vi "variableNames.vi"(11 "pathString":path) -> (2 "spreadsheet string":string, 3 "all rows":string[](array[string]))   [LabVIEW 2017]
uses:
  <userlib>/My Palettes.lib/Files & paths/Spreadsheet/Read From Spreadsheet File (string)-Mod.vi
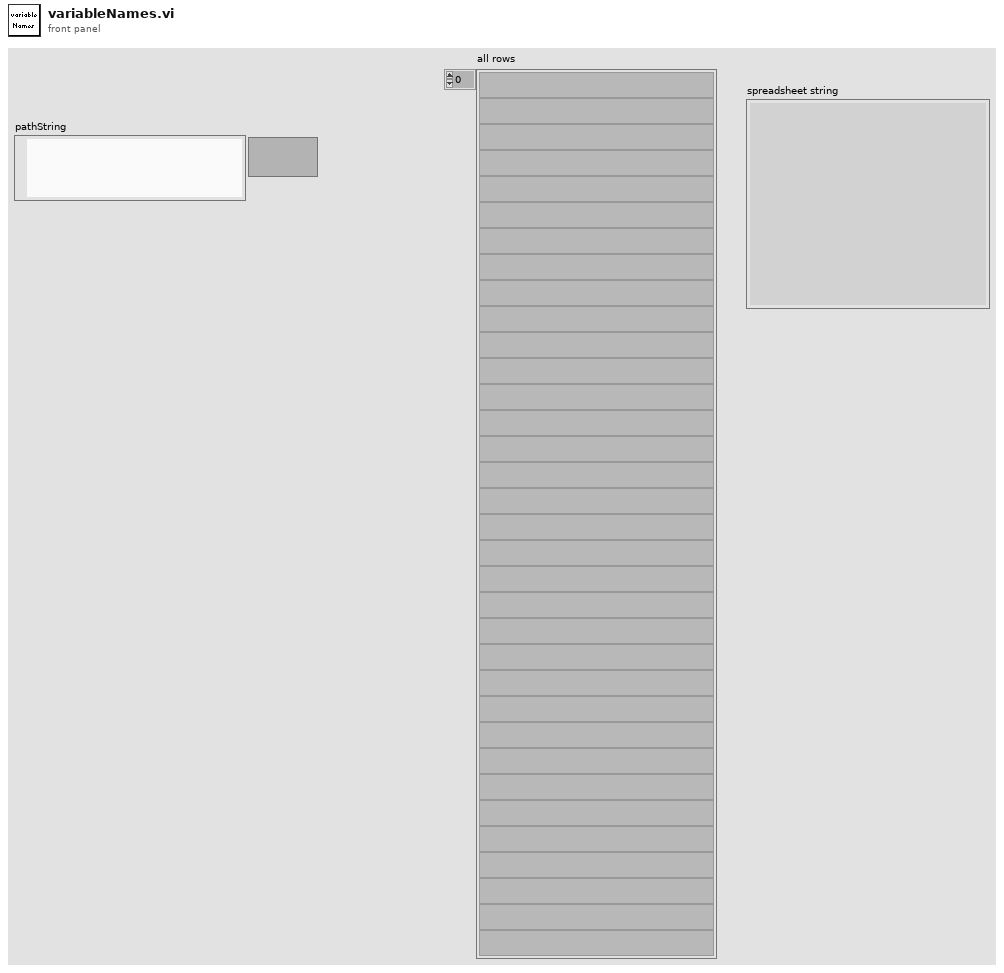
[diagram p1: front panel]
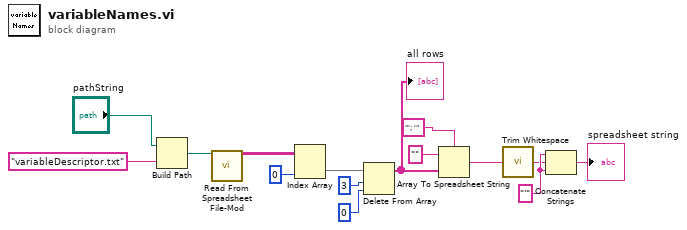
[diagram p0: block diagram]
diagram:
  w5 = "'" ("string")
  n1 = Build Path(base path="pathString", name or relative path="variableDescriptor.txt") -> (appended path=w15:path)
  n2 = call-poly <userlib>:"Read From Spreadsheet File-Mod.vi"("file path (dialog if empty)"=w15) -> ("all rows"=w1:string[][])  [unwired: 9 in, 5 out]
  n3 = Index Array(array=w1, index (col)=0 ("disabled index (col)")) -> (element=w11:string[])  [unwired: 1 in]
  n4 = Delete From Array(array=w11, length=3, index=0) -> (array with subset deleted=w7:string[])  [unwired: 1 out]
  "all rows" <- w7
  n5 = Array To Spreadsheet String(delimiter (Tab)="'; '", array=w7, 3:"" ("format string")) -> (spreadsheet string=w3:string)
  n6 = call <vilib>:"Trim Whitespace.vi"("string"=w3) -> ("trimmed string"=w2:string)  [unwired: 1 in]
  n7 = Concatenate Strings(w5, w2, w5) -> (→"spreadsheet string":string)
